vi "All Modes - Single Module.vi"() -> ()   [LabVIEW 2020, in "BCI-1553 RealTime API Examples.lvlib"]
uses:
  BCI-1553 RealTime API Examples.lvlib
  TypeDefs/Control.ctl
  src/RealTime/Frames & Messages/TypeDefs/Command Type.ctl
  src/RealTime/Frames & Messages/TypeDefs/Command Terminal Address.ctl
  src/RealTime/Frames & Messages/TypeDefs/Command SubAddress.ctl
  src/RealTime/1553 Session/1553 Session.lvclass/1553 Session.ctl
  src/RealTime/1553 Component/1553 Component.lvclass/1553 Component.ctl
  5969a701-9647-44f1-b299-7744b950ea80.vi
  src/RealTime/1553 Component/1553 Component.lvclass
  src/RealTime/1553 SubComponent/1553 SubComponent.lvclass
  src/RealTime/Frames & Messages/Async Message/Async Message.lvclass
  src/RealTime/1553 Session/1553 Session.lvclass
  src/RealTime/Dependencies/FPGA Interface/FPGA Interface.lvclass
  <vilib>/rvi/interface/nirviOpenFPGA/nirviOpenFPGA.xnode
  Bitfiles/BCI-1553-FPGAMain.lvbitx
  FPGA/FPGA Main.vi
  <vilib>/FPGAPlugInAG/cRIO-9030/niLvFpga_Open_cRIO-9030.vi
  <vilib>/rvi/interface/common/dynamic/niFpgaDynamicAddResources.vi
  src/RealTime/BCI-1553 API.lvlib
panel:
  in  "Async Rx Float":dbl=12.0 min=-11.0 max=12.0 step=0.1
  in  "Async Rx Bool":bool
  in  "SubAddress":T1=enum."1"
  in  "Terminal Address":T2=enum."8"
  in  "Async Command Type":T3
  out "Bus A Monitor Log":i32(listbox)
  in  "Sourcing Scaled Data":dbl[](array[numeric])=[1.0, 2.5, 0.0, 1214.2, 1.0, 400.9, 1.0, 7.1]
  in  "Sourcing Parameters":string[](array[string])=["RT8TxSA1Boolean", "RT8TxSA1Float", "RT8TxSA2Boolean", "RT8TxSA2Float", "RT16TxSA1Boolean", "RT16TxSA1Float", "RT16TxSA2Boolean", "RT16TxSA2Float"]
  out "Scaled Data":dbl[](array[numeric])
  out "Sinking Parameters":string[](array[string])
  in  "Example Control":T4
  # "BCI-1553 RealTime API Example"
  # "Idle Sinking Data"
  # "Quick Start:\n\n1. Press the run button.\n2. Run the 'Update Data' case\n3. Start sending Async Messages\n4. Read the Bus Monitor Log to validate transactions"
  # "How to use this example:\n\n1. Make sure the FPGA is setup correctly. This code relies a bitfile being deployed to a specific path on the target. If preferred, the initialization can be update to use the FPGA refnum instead (See the diagram disable structure).\n\n2. Press the run arrow and make sure there are no errors generated during initialization or deployment.\n\nIdle: All the sinking parameters in the session are read. For the bus contoller, this is transmit parameters. For the remote terminals, this is receive parameters.\n\nUpdate Data: Updates any sourcing parameters in the session. In this case, it is already configured to update the values stored for the transmit commands on the remote terminals. This could be extended to update other sourcing values as well, such as receive commands on a bus controller.\n\nSend Async Message: Sends an asynchronous command out on the bus. The Async command can be configured for transmit or receive. When configured for receive, you can adjust the values being transmitted via the async command. When sent as a transmit command, the Idle Data should update shortly with parameters representing the transmitted values.\n\nRead Bus Monitor Log: Reads all the traffic tha has been transacted across Bus A. The data stored byt he BCI-1553 Bus Monitor will eventually roll-over, so it is up to the developer to handle reading the buffer frequently enough to detect all data tranactions and to store the logs. For ease of transaction out of the RealTime layer, there is a VI available to retrieve an encoded raw copy of the Bus Monitor log in the API.\n\nStart/Stop <SubComponent>: Starts or stops a particular SubComponent. This can be used to stop the operation of one SubComponent, while keeping the others running. Similarly, it can be used to stop Subcomponents that are no longer necessary.\n\nStop Example: Stops all the BCI-1553 devices on the bus and shuts down the session.\n\nOther notes:\n\nRT 1 Address: 08\nValid SubAddresses: Tx01, Tx02, Rx01, Rx02\n\nRT 2 Address: 16\nValid SubAddresses: Tx01, Tx02, Rx01, Rx02\n\nPlease read through the block diagram documentation for more information on how the API is used to setup this session."
  # "Async Messaging"
  # "Note:\n\nThe Remote Terminals are at addresses\n8 and 16. There are transmit and receive\ncommands setup for SubAddresses 1 and 2.\n\nAny Asynchronous messages sent outside of this specification should exhibit no-response behavior."
  # "Update Sourcing Data"
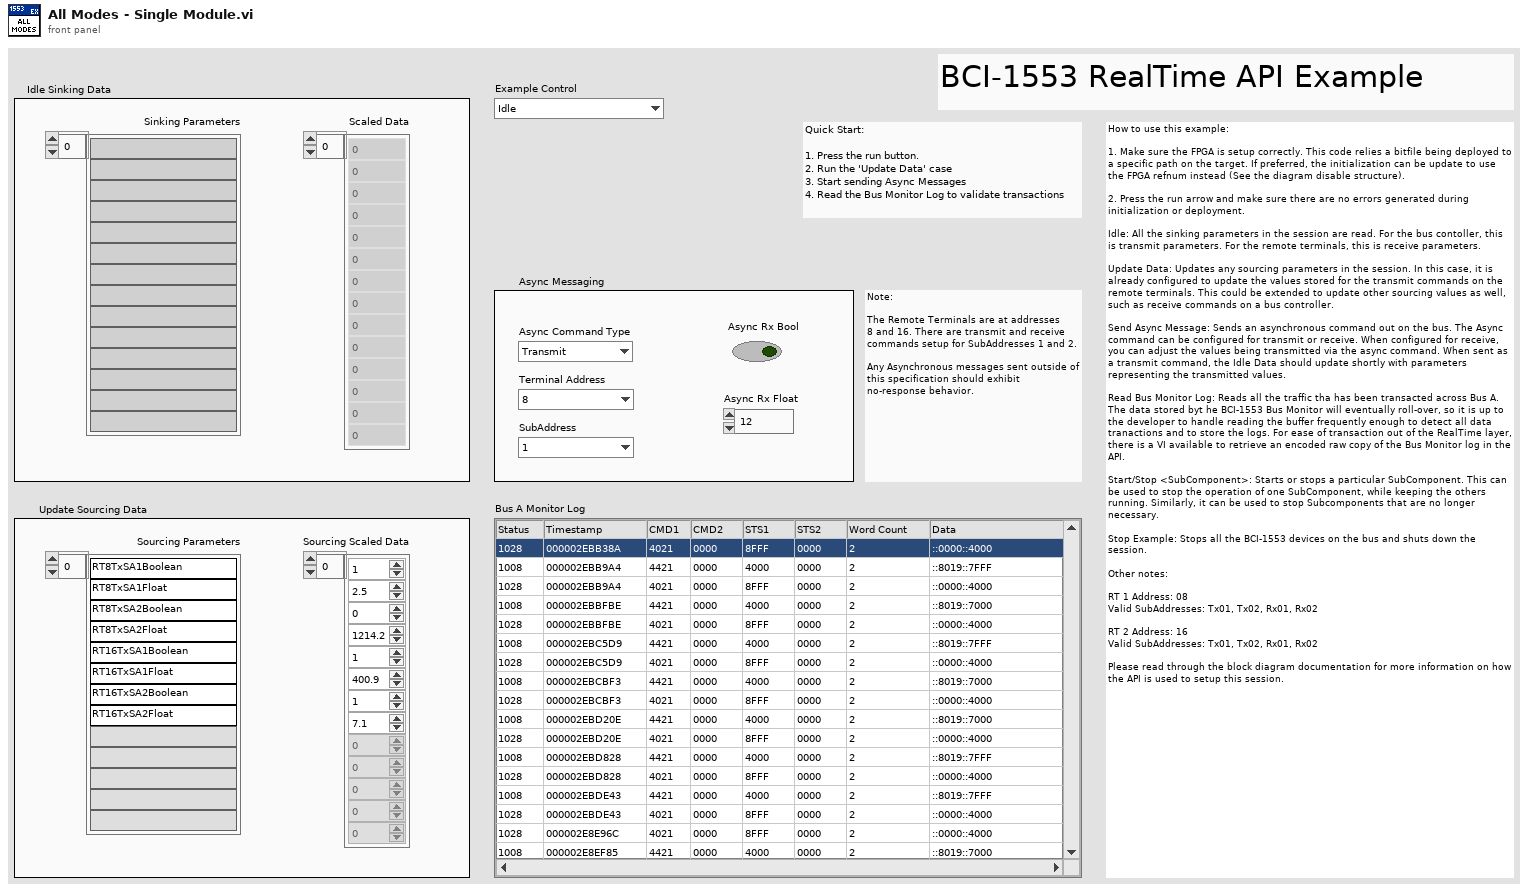
[diagram p1: front panel]
types:
  T1 = typedef "BCI-1553 API.lvlib/Command SubAddress.ctl" = enum16{"Mode Code", "1", "2", "3", "4", "5", "6", "7", "8", "9", "10", "11", "12", "13", "14", "15", "16", "17", "18", "19", "20", "21", "22", "23", "24", "25", "26", "27", "28", "29", "30"}
  T2 = typedef "BCI-1553 API.lvlib/Command Terminal Address.ctl" = enum16{"0", "1", "2", "3", "4", "5", "6", "7", "8", "9", "10", "11", "12", "13", "14", "15", "16", "17", "18", "19", "20", "21", "22", "23", "24", "25", "26", "27", "28", "29", "30", "Broadcast"}
  T3 = typedef "BCI-1553 API.lvlib/Command Type.ctl" = enum16{"Transmit", "Receive"}
  T4 = typedef "BCI-1553 RealTime API Examples.lvlib/Control.ctl" = enum16{"Idle", "Update Data", "Start Bus Controller", "Stop Bus Controller", "Send Async Message", "Start Remote Terminal 1", "Stop Remote Terminal 1", "Start Remote Terminal 2", "Stop Remote Terminal 2", "Read Bus Monitor Log", "Stop Example"}
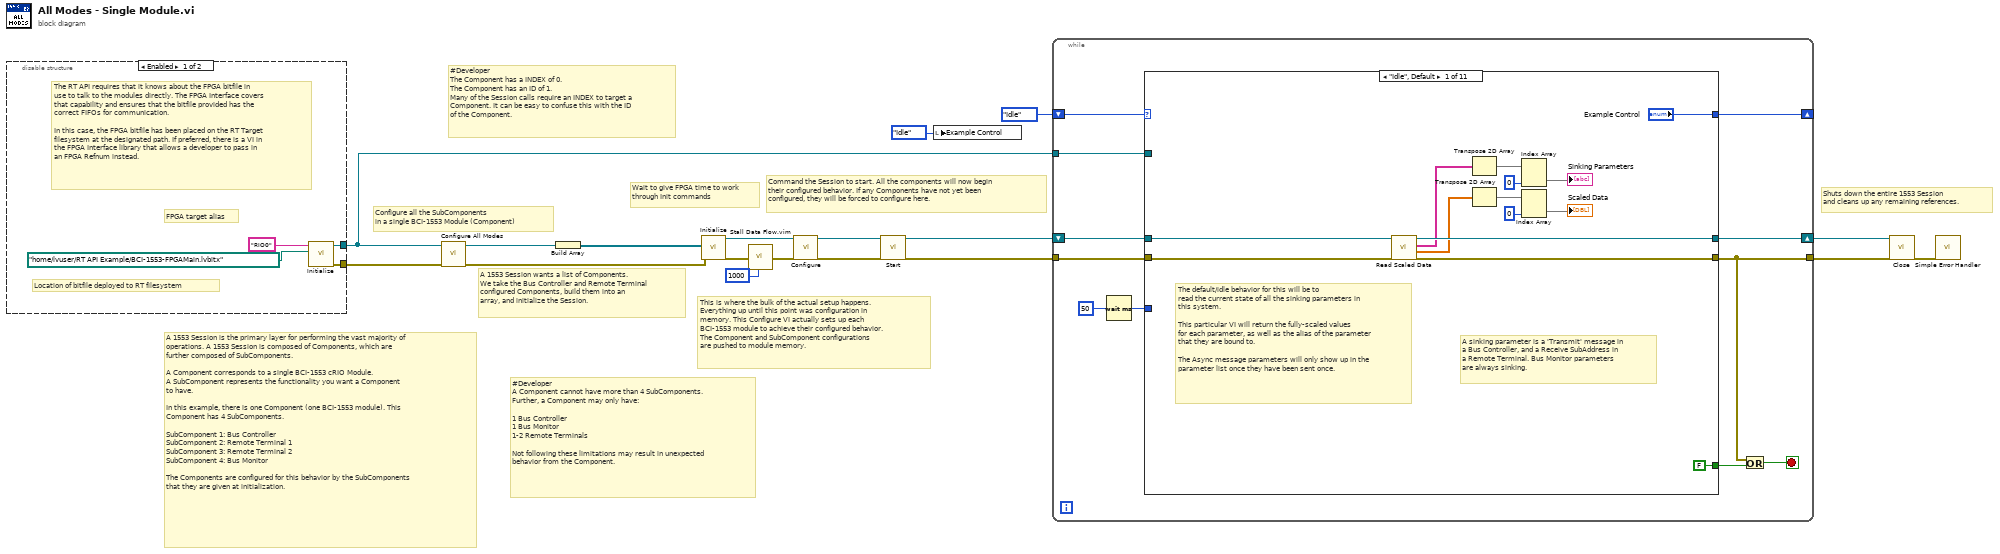
[diagram p0: block diagram]
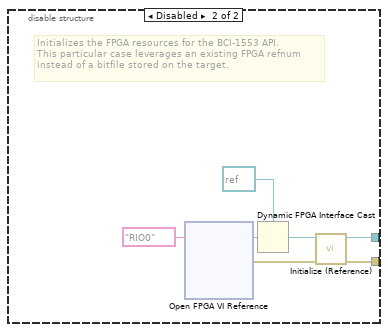
[diagram p2: hidden frame]
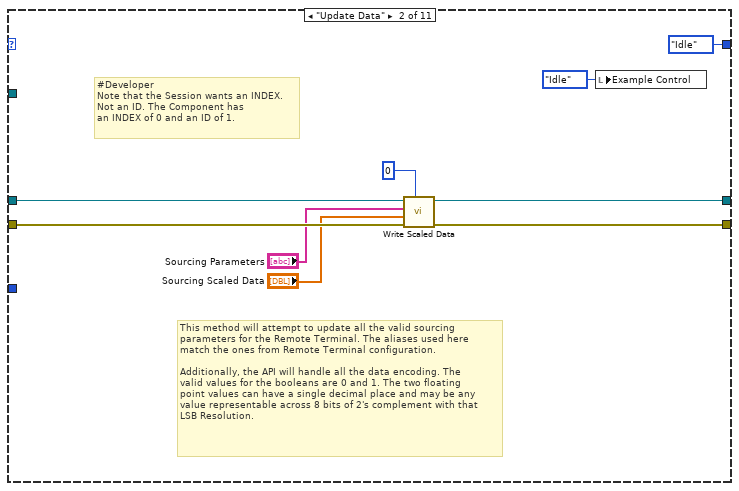
[diagram p3: hidden frame]
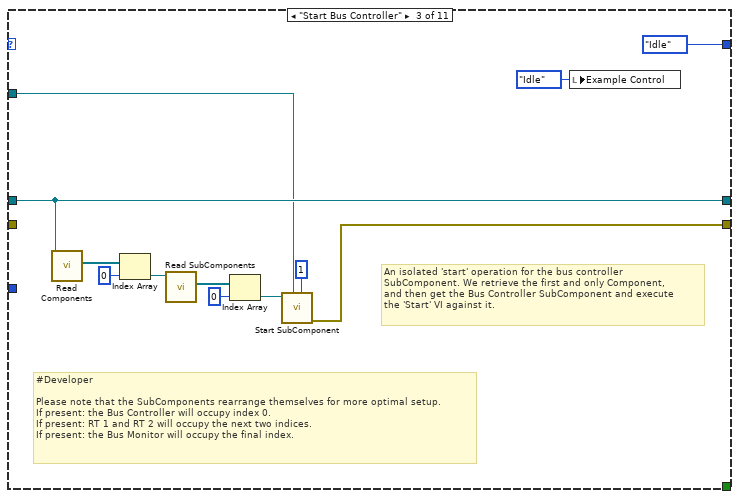
[diagram p4: hidden frame]
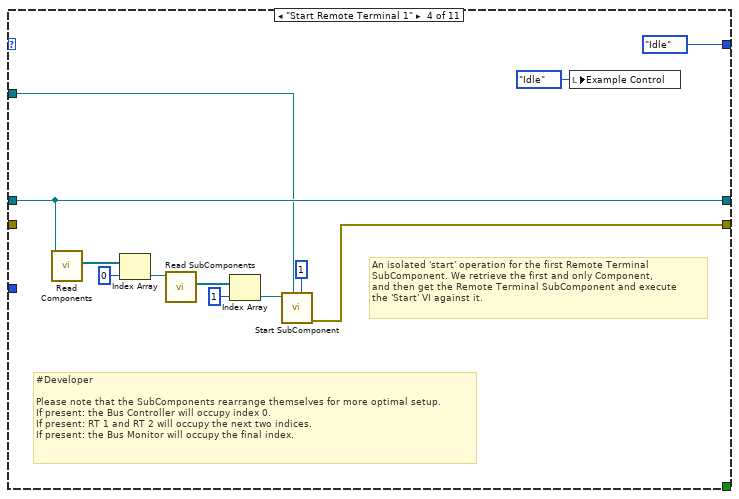
[diagram p5: hidden frame]
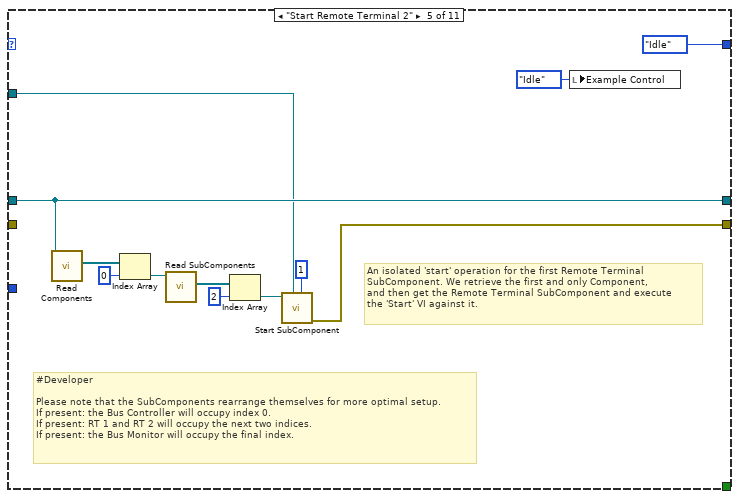
[diagram p6: hidden frame]
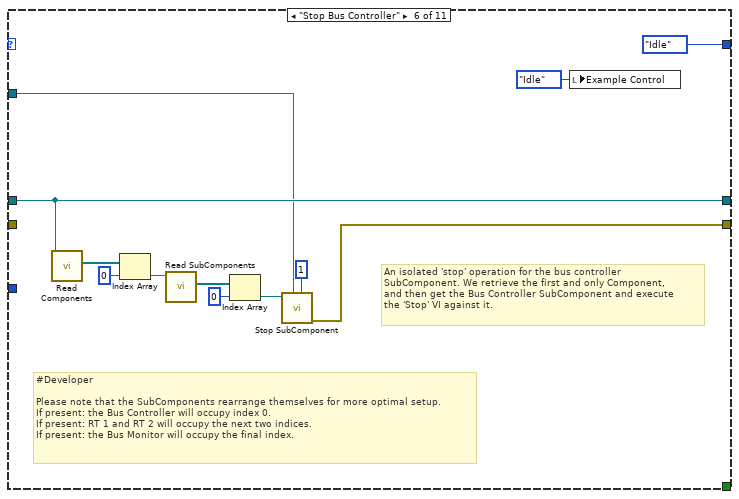
[diagram p7: hidden frame]
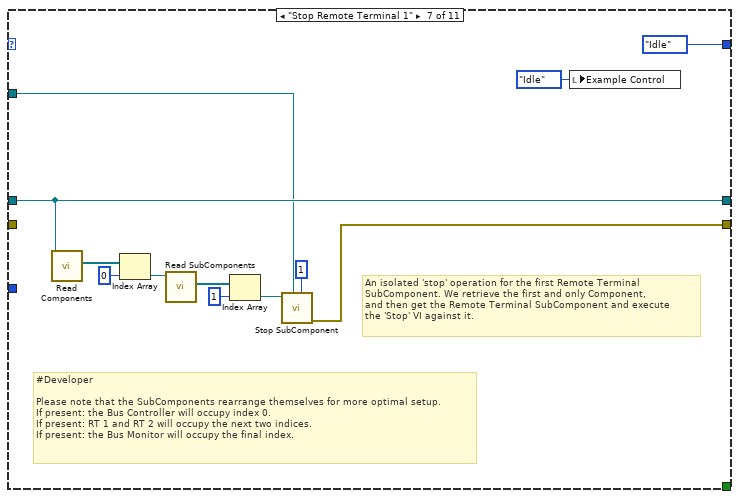
[diagram p8: hidden frame]
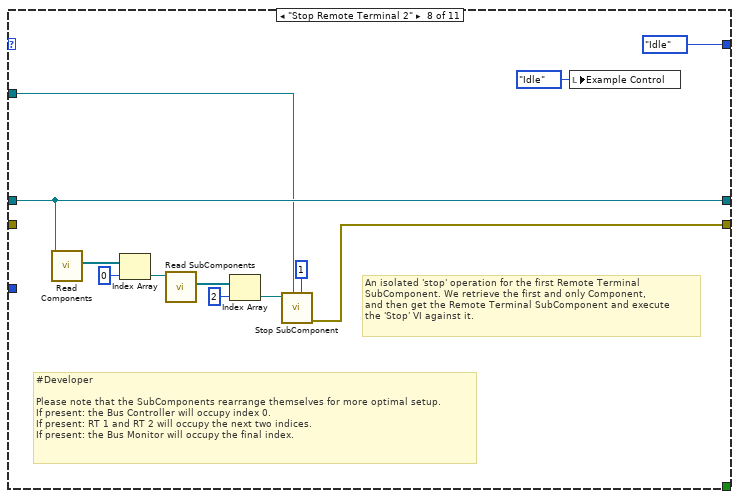
[diagram p9: hidden frame]
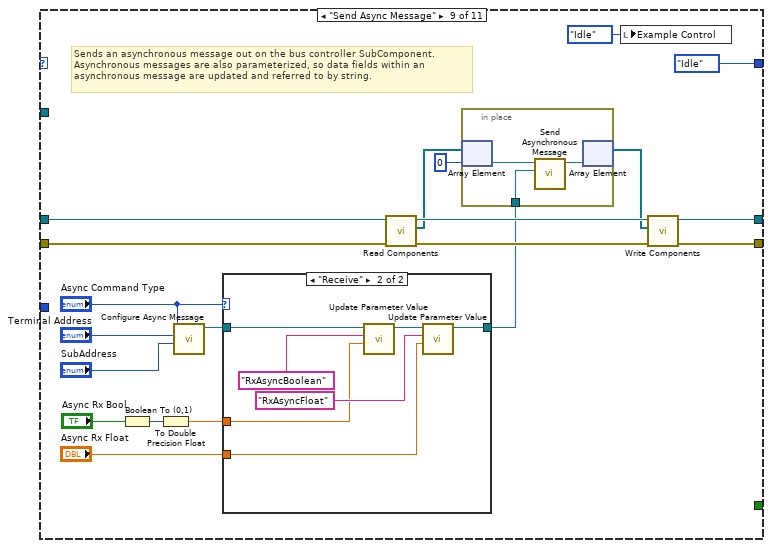
[diagram p10: hidden frame]
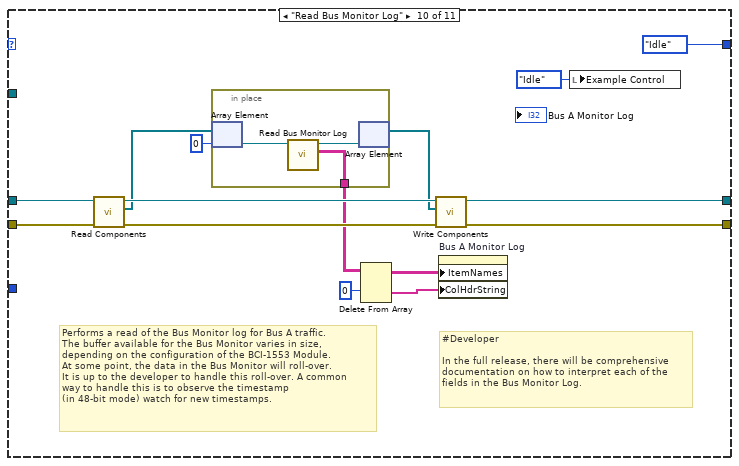
[diagram p12: hidden frame]
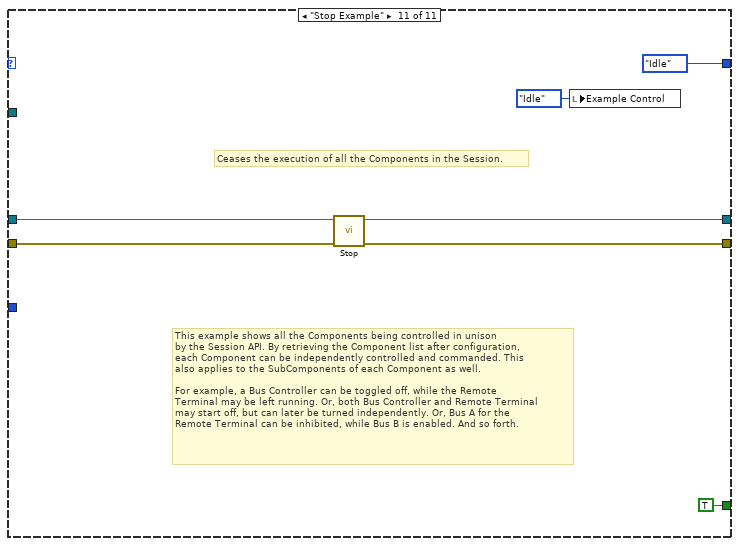
[diagram p13: hidden frame]
diagram:
  # "Wait to give FPGA time to work through Init commands"
  # "#Developer\nThe Component has a INDEX of 0.\nThe Component has an ID of 1.\nMany of the Session calls require an INDEX to target a\nComponent. It can be easy to confuse this with the ID\nof the Component."
  # "#Developer\nA Component cannot have more than 4 SubComponents.\nFurther, a Component may only have:\n\n1 Bus Controller\n1 Bus Monitor\n1-2 Remote Terminals\n\nNot following these limitations may result in unexpected\nbehavior from the Component."
  # "Shuts down the entire 1553 Session\nand cleans up any remaining references."
  # "Command the Session to start. All the components will now begin\ntheir configured behavior. If any Components have not yet been \nconfigured, they will be forced to configure here."
  # "This is where the bulk of the actual setup happens.\nEverything up until this point was configuration in\nmemory. This Configure VI actually sets up each \nBCI-1553 module to achieve their configured behavior.\nThe Component and SubComponent configurations\nare pushed to module memory."
  # "A 1553 Session wants a list of Components.\nWe take the Bus Controller and Remote Terminal\nconfigured Components, build them into an\narray, and initialize the Session."
  # "Configure all the SubComponents\nin a single BCI-1553 Module (Component)"
  # "A 1553 Session is the primary layer for performing the vast majority of\noperations. A 1553 Session is composed of Components, which are \nfurther composed of SubComponents.\n\nA Component corresponds to a single BCI-1553 cRIO Module.\nA SubComponent represents the functionality you want a Component\nto have.\n\nIn this example, there is one Component (one BCI-1553 module). This \nComponent has 4 SubComponents.\n\nSubComponent 1: Bus Controller\nSubComponent 2: Remote Terminal 1\nSubComponent 3: Remote Terminal 2\nSubComponent 4: Bus Monitor\n\nThe Components are configured for this behavior by the SubComponents\nthat they are given at initialization."
  n1 = disable-structure shown="Enabled" {
    disable-tunnel: [w22 w28] -> w18
    disable-tunnel: [w21 w29] -> w5
    frame Enabled {
      # "The RT API requires that it knows about the FPGA bitfile in\nuse to talk to the modules directly. The FPGA Interface covers\nthat capability and ensures that the bitfile provided has the\ncorrect FIFOs for communication.\n\nIn this case, the FPGA bitfile has been placed on the RT Target\nfilesystem at the designated path. If preferred, there is a VI in\nthe FPGA Interface library that allows a developer to pass in\nan FPGA Refnum instead."
      # "Location of bitfile deployed to RT filesystem"
      # "FPGA target alias"
      n2 = call "Initialize.vi"("Bitfile path"=path "/home/lvuser/RT API Example/BCI-1553-FPGAMain.lvbitx", "Device address"="RIO0") -> ("error out"=w22:errorcluster, "FPGA Interface out"=w21:refnum<class "FPGA Interface.lvclass">)  [unwired: 8 in]
    }
    frame Disabled {
      # "Initializes the FPGA resources for the BCI-1553 API.\nThis particular case leverages an existing FPGA refnum\ninstead of a bitfile stored on the target."
      n3 = xnode "Open FPGA VI Reference"("resource name"=tag "RIO0") -> ("FPGA VI Reference Out"=w27:refnum<k20>, "error out"=w24:errorcluster)  [unwired: 1 in]
      n4 = Dynamic FPGA Interface Cast(Session In=refnum<k20> refnum ("FPGA Refnum"), Type=w27) -> (Session Out=w25:refnum<k20>)
      n5 = call "Initialize (Reference).vi"("error in (no error)"=w24, "FPGA Refnum"=w25) -> ("error out"=w28:errorcluster, "FPGA Interface out"=w29:refnum<class "FPGA Interface.lvclass">)  [unwired: 8 in]
    }
  }
  n6 = call "Configure All Modes.vi"("error in (no error)"=w18, "FPGA Interface"=w5) -> ("error out"=w15:errorcluster, "1553 Component"=w17:refnum<class "1553 Component.lvclass">)  [unwired: 8 in]
  n7 = Build Array(w17) -> (w16:refnum<class "1553 Component.lvclass">[])
  n8 = call "Initialize.vi"("error in (no error)"=w15, "Components"=w16) -> ("error out"=w3:errorcluster, "1553 Board out"=w14:refnum<class "1553 Session.lvclass">)  [unwired: 8 in]
  n9 = call "Stall Data Flow.vim"("value in"=w3, "milliseconds to wait"=u32 1000) -> ("value out"=w2:errorcluster)  [unwired: 1 out]
  n10 = call-dynamic "Configure.vi"("error in (no error)"=w2, "1553 Board in"=w14) -> ("error out"=w12:errorcluster, "1553 Board out"=w13:refnum<class "1553 Session.lvclass">)  [unwired: 8 in]
  n11 = call-dynamic "Start.vi"("error in (no error)"=w12, "1553 Board in"=w13) -> ("error out"=w10:errorcluster, "1553 Board out"=w11:refnum<class "1553 Session.lvclass">)  [unwired: 8 in]
  n12 = local write "Example Control"(Control."Idle" ("Example Control")) -> ()
  n13 = while {
    shift-right: [w38] -> w7
    shift-left: w11 -> [w37]
    tunnel: w10 -> [w36]
    shift-right: [w39] -> _
    shift-left: Control."Idle" ("Example Control") -> [w40]
    tunnel: [w30] -> w6
    tunnel: w5 -> [w33]
    stop <- w31 stop-if-true
    n14 = Wait (ms)(milliseconds to wait=u32 50) -> (millisecond timer value=w34:u32)
    n15 = case shown="\"Idle\", Default" w40 {
      tunnel: [FALSE _ _ _ _ _ _ _ _ _ TRUE] -> w32
      tunnel: ["Example Control" Control."Idle" ("Example Control") Control."Idle" ("Example Control") Control."Idle" ("Example Control") Control."Idle" ("Example Control") Control."Idle" ("Example Control") Control."Idle" ("Example Control") Control."Idle" ("Example Control") Control."Idle" ("Example Control") Control."Idle" ("Example Control") Control."Idle" ("Example Control")] -> w39
      tunnel: [w51 w60 w73 w85 w97 w109 w121 w133 w147 w176 w188] -> w38
      tunnel: w37 -> [w52 w61 w73 w85 w97 w109 w121 w133 w148 w178 w189]
      tunnel: [w49 w58 w64 w76 w88 w100 w112 w124 w145 w174 w186] -> w30
      tunnel: w36 -> [w50 w59 _ _ _ _ _ _ w146 w179 w187]
      tunnel: w34 -> [_ _ _ _ _ _ _ _ _ _ _]
      tunnel: w33 -> [_ _ w65 w77 w89 w101 w113 w125 _ _ _]
      frame "Idle", Default {
        # "A sinking parameter is a 'Transmit' message in\na Bus Controller, and a Receive SubAddress in\na Remote Terminal. Bus Monitor parameters\nare always sinking."
        # "The default/idle behavior for this will be to \nread the current state of all the sinking parameters in \nthis system.\n\nThis particular VI will return the fully-scaled values\nfor each parameter, as well as the alias of the parameter\nthat they are bound to.\n\nThe Async message parameters will only show up in the\nparameter list once they have been sent once."
        n16 = call-dynamic "Read Scaled Data.vi"("error in (no error)"=w50, "1553 Board in"=w52) -> ("error out"=w49:errorcluster, "Scaled Data"=w47:dbl[][], "Parameters"=w48:string[][], "1553 Board out"=w51:refnum<class "1553 Session.lvclass">)  [unwired: 6 in]
        n17 = Transpose 2D Array(2D array=w48) -> (transposed array=w46:string[][])
        n18 = Transpose 2D Array(2D array=w47) -> (transposed array=w42:dbl[][])
        n19 = Index Array(array=w46, index (col)=0 ("disabled index (col)")) -> (element=→"Sinking Parameters":string[])  [unwired: 1 in]
        n20 = Index Array(array=w42, index (col)=0 ("disabled index (col)")) -> (element=→"Scaled Data":dbl[])  [unwired: 1 in]
      }
      frame "Update Data" {
        # "This method will attempt to update all the valid sourcing\nparameters for the Remote Terminal. The aliases used here\nmatch the ones from Remote Terminal configuration.\n\nAdditionally, the API will handle all the data encoding. The\nvalid values for the booleans are 0 and 1. The two floating \npoint values can have a single decimal place and may be any\nvalue representable across 8 bits of 2's complement with that\nLSB Resolution."
        # "#Developer\nNote that the Session wants an INDEX.\nNot an ID. The Component has\nan INDEX of 0 and an ID of 1."
        n21 = call-dynamic "Write Scaled Data.vi"("Component Index"=0, "error in (no error)"=w59, "Scaled Data"="Sourcing Scaled Data", "Parameters"="Sourcing Parameters", "1553 Board in"=w61) -> ("error out"=w58:errorcluster, "1553 Board out"=w60:refnum<class "1553 Session.lvclass">)  [unwired: 5 in]
        n22 = local write "Example Control"(Control."Idle" ("Example Control")) -> ()
      }
      frame "Start Bus Controller" {
        # "#Developer\n\nPlease note that the SubComponents rearrange themselves for more optimal setup.\nIf present: the Bus Controller will occupy index 0.\nIf present: RT 1 and RT 2 will occupy the next two indices.\nIf present: the Bus Monitor will occupy the final index."
        # "An isolated 'start' operation for the bus controller\nSubComponent. We retrieve the first and only Component,\nand then get the Bus Controller SubComponent and execute\nthe 'Start' VI against it."
        n23 = call "Read Components.vi"("1553 Board in"=w73) -> ("Components"=w72:refnum<class "1553 Component.lvclass">[])  [unwired: 8 in, 2 out]
        n24 = Index Array(array=w72, index=0) -> (element=w70:refnum<class "1553 Component.lvclass">)
        n25 = call "Read SubComponents.vi"("1553 Component in"=w70) -> ("SubComponents"=w68:refnum<class "1553 SubComponent.lvclass">[])  [unwired: 8 in, 2 out]
        n26 = Index Array(array=w68, index=0) -> (element=w67:refnum<class "1553 SubComponent.lvclass">)
        n27 = call-dynamic "Start SubComponent.vi"("Component ID"=u8 1, "FPGA Interface"=w65, "1553 SubComponent in"=w67) -> ("error out"=w64:errorcluster)  [unwired: 7 in, 1 out]
        n28 = local write "Example Control"(Control."Idle" ("Example Control")) -> ()
      }
      frame "Start Remote Terminal 1" {
        # "#Developer\n\nPlease note that the SubComponents rearrange themselves for more optimal setup.\nIf present: the Bus Controller will occupy index 0.\nIf present: RT 1 and RT 2 will occupy the next two indices.\nIf present: the Bus Monitor will occupy the final index."
        # "An isolated 'start' operation for the first Remote Terminal\nSubComponent. We retrieve the first and only Component,\nand then get the Remote Terminal SubComponent and execute\nthe 'Start' VI against it."
        n29 = call "Read Components.vi"("1553 Board in"=w85) -> ("Components"=w84:refnum<class "1553 Component.lvclass">[])  [unwired: 8 in, 2 out]
        n30 = Index Array(array=w84, index=0) -> (element=w82:refnum<class "1553 Component.lvclass">)
        n31 = call "Read SubComponents.vi"("1553 Component in"=w82) -> ("SubComponents"=w80:refnum<class "1553 SubComponent.lvclass">[])  [unwired: 8 in, 2 out]
        n32 = Index Array(array=w80, index=1) -> (element=w79:refnum<class "1553 SubComponent.lvclass">)
        n33 = call-dynamic "Start SubComponent.vi"("Component ID"=u8 1, "FPGA Interface"=w77, "1553 SubComponent in"=w79) -> ("error out"=w76:errorcluster)  [unwired: 7 in, 1 out]
        n34 = local write "Example Control"(Control."Idle" ("Example Control")) -> ()
      }
      frame "Start Remote Terminal 2" {
        # "An isolated 'start' operation for the first Remote Terminal\nSubComponent. We retrieve the first and only Component,\nand then get the Remote Terminal SubComponent and execute\nthe 'Start' VI against it."
        # "#Developer\n\nPlease note that the SubComponents rearrange themselves for more optimal setup.\nIf present: the Bus Controller will occupy index 0.\nIf present: RT 1 and RT 2 will occupy the next two indices.\nIf present: the Bus Monitor will occupy the final index."
        n35 = call "Read Components.vi"("1553 Board in"=w97) -> ("Components"=w96:refnum<class "1553 Component.lvclass">[])  [unwired: 8 in, 2 out]
        n36 = Index Array(array=w96, index=0) -> (element=w94:refnum<class "1553 Component.lvclass">)
        n37 = call "Read SubComponents.vi"("1553 Component in"=w94) -> ("SubComponents"=w92:refnum<class "1553 SubComponent.lvclass">[])  [unwired: 8 in, 2 out]
        n38 = Index Array(array=w92, index=2) -> (element=w91:refnum<class "1553 SubComponent.lvclass">)
        n39 = call-dynamic "Start SubComponent.vi"("Component ID"=u8 1, "FPGA Interface"=w89, "1553 SubComponent in"=w91) -> ("error out"=w88:errorcluster)  [unwired: 7 in, 1 out]
        n40 = local write "Example Control"(Control."Idle" ("Example Control")) -> ()
      }
      frame "Stop Bus Controller" {
        # "#Developer\n\nPlease note that the SubComponents rearrange themselves for more optimal setup.\nIf present: the Bus Controller will occupy index 0.\nIf present: RT 1 and RT 2 will occupy the next two indices.\nIf present: the Bus Monitor will occupy the final index."
        # "An isolated 'stop' operation for the bus controller\nSubComponent. We retrieve the first and only Component,\nand then get the Bus Controller SubComponent and execute\nthe 'Stop' VI against it."
        n41 = call "Read Components.vi"("1553 Board in"=w109) -> ("Components"=w108:refnum<class "1553 Component.lvclass">[])  [unwired: 8 in, 2 out]
        n42 = Index Array(array=w108, index=0) -> (element=w106:refnum<class "1553 Component.lvclass">)
        n43 = call "Read SubComponents.vi"("1553 Component in"=w106) -> ("SubComponents"=w104:refnum<class "1553 SubComponent.lvclass">[])  [unwired: 8 in, 2 out]
        n44 = Index Array(array=w104, index=0) -> (element=w103:refnum<class "1553 SubComponent.lvclass">)
        n45 = call-dynamic "Stop SubComponent.vi"("Component ID"=u8 1, "FPGA Interface"=w101, "1553 SubComponent in"=w103) -> ("error out"=w100:errorcluster)  [unwired: 7 in, 1 out]
        n46 = local write "Example Control"(Control."Idle" ("Example Control")) -> ()
      }
      frame "Stop Remote Terminal 1" {
        # "An isolated 'stop' operation for the first Remote Terminal\nSubComponent. We retrieve the first and only Component,\nand then get the Remote Terminal SubComponent and execute\nthe 'Stop' VI against it."
        # "#Developer\n\nPlease note that the SubComponents rearrange themselves for more optimal setup.\nIf present: the Bus Controller will occupy index 0.\nIf present: RT 1 and RT 2 will occupy the next two indices.\nIf present: the Bus Monitor will occupy the final index."
        n47 = call "Read Components.vi"("1553 Board in"=w121) -> ("Components"=w120:refnum<class "1553 Component.lvclass">[])  [unwired: 8 in, 2 out]
        n48 = Index Array(array=w120, index=0) -> (element=w118:refnum<class "1553 Component.lvclass">)
        n49 = call "Read SubComponents.vi"("1553 Component in"=w118) -> ("SubComponents"=w116:refnum<class "1553 SubComponent.lvclass">[])  [unwired: 8 in, 2 out]
        n50 = Index Array(array=w116, index=1) -> (element=w115:refnum<class "1553 SubComponent.lvclass">)
        n51 = call-dynamic "Stop SubComponent.vi"("Component ID"=u8 1, "FPGA Interface"=w113, "1553 SubComponent in"=w115) -> ("error out"=w112:errorcluster)  [unwired: 7 in, 1 out]
        n52 = local write "Example Control"(Control."Idle" ("Example Control")) -> ()
      }
      frame "Stop Remote Terminal 2" {
        # "An isolated 'stop' operation for the first Remote Terminal\nSubComponent. We retrieve the first and only Component,\nand then get the Remote Terminal SubComponent and execute\nthe 'Stop' VI against it."
        # "#Developer\n\nPlease note that the SubComponents rearrange themselves for more optimal setup.\nIf present: the Bus Controller will occupy index 0.\nIf present: RT 1 and RT 2 will occupy the next two indices.\nIf present: the Bus Monitor will occupy the final index."
        n53 = call "Read Components.vi"("1553 Board in"=w133) -> ("Components"=w132:refnum<class "1553 Component.lvclass">[])  [unwired: 8 in, 2 out]
        n54 = Index Array(array=w132, index=0) -> (element=w130:refnum<class "1553 Component.lvclass">)
        n55 = call "Read SubComponents.vi"("1553 Component in"=w130) -> ("SubComponents"=w128:refnum<class "1553 SubComponent.lvclass">[])  [unwired: 8 in, 2 out]
        n56 = Index Array(array=w128, index=2) -> (element=w127:refnum<class "1553 SubComponent.lvclass">)
        n57 = call-dynamic "Stop SubComponent.vi"("Component ID"=u8 1, "FPGA Interface"=w125, "1553 SubComponent in"=w127) -> ("error out"=w124:errorcluster)  [unwired: 7 in, 1 out]
        n58 = local write "Example Control"(Control."Idle" ("Example Control")) -> ()
      }
      frame "Send Async Message" {
        # "Sends an asynchronous message out on the bus controller SubComponent.\nAsynchronous messages are also parameterized, so data fields within an\nasynchronous message are updated and referred to by string."
        n59 = Boolean To (0,1)(Boolean="Async Rx Bool") -> (0, 1=w138:i16)
        n60 = To Double Precision Float(number=w138) -> (double precision float=w136:dbl)
        n61 = call "Configure Async Message.vi"("SubAddress"="SubAddress", "Terminal Address"="Terminal Address", "Async Command Type"="Async Command Type") -> ("Async Message"=w142:refnum<class "Async Message.lvclass">)  [unwired: 8 in]
        n62 = case shown="\"Receive\"" "Async Command Type" {
          tunnel: w142 -> [w156 w163]
          tunnel: [w156 w159] -> w140
          tunnel: "Async Rx Float" -> [_ w158]
          tunnel: w136 -> [_ w157]
          frame "Transmit", Default {
          }
          frame "Receive" {
            n63 = call-dynamic "Update Parameter Value.vi"("Value"=w157, "Parameter"="RxAsyncBoolean" ("Parameter Name"), "Async Message in"=w163) -> ("Async Message out"=w162:refnum<class "Async Message.lvclass">)  [unwired: 7 in, 1 out]
            n64 = call-dynamic "Update Parameter Value.vi"("Value"=w158, "Parameter"="RxAsyncFloat" ("Parameter Name"), "Async Message in"=w162) -> ("Async Message out"=w159:refnum<class "Async Message.lvclass">)  [unwired: 7 in, 1 out]
          }
        }
        n65 = call "Read Components.vi"("error in (no error)"=w146, "1553 Board in"=w148) -> ("error out"=w152:errorcluster, "Components"=w151:refnum<class "1553 Component.lvclass">[], "1553 Board out"=w153:refnum<class "1553 Session.lvclass">)  [unwired: 7 in]
        n66 = in-place {
          in-place-border: w140 -> [w164]
          n67 = in-place-array #1(w151, 0) -> (w166:refnum<class "1553 Component.lvclass">)
          n68 = call-dynamic "Send Asynchronous Message.vi"("Async Message"=w164, "1553 Component in"=w166) -> ("1553 Component out"=w165:refnum<class "1553 Component.lvclass">)  [unwired: 8 in, 1 out]
          n69 = in-place-array #1(w165) -> (w149:refnum<class "1553 Component.lvclass">[])  [unwired: 1 out]
        }
        n70 = local write "Example Control"(Control."Idle" ("Example Control")) -> ()
        n71 = call "Write Components.vi"("error in (no error)"=w152, "Components"=w149, "1553 Board in"=w153) -> ("error out"=w145:errorcluster, "1553 Board out"=w147:refnum<class "1553 Session.lvclass">)  [unwired: 7 in]
      }
      frame "Read Bus Monitor Log" {
        # "#Developer\n\nIn the full release, there will be comprehensive\ndocumentation on how to interpret each of the\nfields in the Bus Monitor Log."
        # "Performs a read of the Bus Monitor log for Bus A traffic.\nThe buffer available for the Bus Monitor varies in size,\ndepending on the configuration of the BCI-1553 Module.\nAt some point, the data in the Bus Monitor will roll-over.\nIt is up to the developer to handle this roll-over. A common\nway to handle this is to observe the timestamp\n(in 48-bit mode) watch for new timestamps."
        n72 = call "Read Components.vi"("error in (no error)"=w179, "1553 Board in"=w178) -> ("error out"=w175:errorcluster, "Components"=w173:refnum<class "1553 Component.lvclass">[], "1553 Board out"=w177:refnum<class "1553 Session.lvclass">)  [unwired: 7 in]
        n73 = in-place {
          in-place-border: [w182] -> w169
          n74 = in-place-array #2(w173, 0) -> (w184:refnum<class "1553 Component.lvclass">)
          n75 = call-dynamic "Read Bus Monitor Log.vi"("1553 Component in"=w184) -> ("Bus A Monitor Log"=w182:string[][], "1553 Component out"=w183:refnum<class "1553 Component.lvclass">)  [unwired: 7 in, 2 out]
          n76 = in-place-array #2(w183) -> (w171:refnum<class "1553 Component.lvclass">[])  [unwired: 1 out]
        }
        n77 = Delete From Array(array=w169, index (row)=0) -> (deleted portion=w167:string[], array with subset deleted=w168:string[][])  [unwired: 2 in]
        n78 = call "Write Components.vi"("error in (no error)"=w175, "Components"=w171, "1553 Board in"=w177) -> ("error out"=w174:errorcluster, "1553 Board out"=w176:refnum<class "1553 Session.lvclass">)  [unwired: 7 in]
        n79 = property on="Bus A Monitor Log" class="MCListbox (strict)"("ItemNames"=w168, "ColHdrString"=w167) -> ()  [unwired: 2 in, 2 out]
        n80 = local write "Example Control"(Control."Idle" ("Example Control")) -> ()
      }
      frame "Stop Example" {
        # "This example shows all the Components being controlled in unison\nby the Session API. By retrieving the Component list after configuration,\neach Component can be independently controlled and commanded. This\nalso applies to the SubComponents of each Component as well.\n\nFor example, a Bus Controller can be toggled off, while the Remote\nTerminal may be left running. Or, both Bus Controller and Remote Terminal\nmay start off, but can later be turned independently. Or, Bus A for the \nRemote Terminal can be inhibited, while Bus B is enabled. And so forth."
        # "Ceases the execution of all the Components in the Session."
        n81 = call-dynamic "Stop.vi"("error in (no error)"=w187, "1553 Board in"=w189) -> ("error out"=w186:errorcluster, "1553 Board out"=w188:refnum<class "1553 Session.lvclass">)  [unwired: 8 in]
        n82 = local write "Example Control"(Control."Idle" ("Example Control")) -> ()
      }
    }
    n83 = Or(x=w30, y=w32) -> (x .or. y?=w31:bool)
  }
  n84 = call-dynamic "Close.vi"("error in (no error)"=w6, "1553 Board in"=w7) -> ("error out"=w4:errorcluster)  [unwired: 9 in]
  n85 = call <vilib>:"Simple Error Handler.vi"("error in (no error)"=w4) -> ()  [unwired: 4 in, 5 out]
